vi "visadenemesi_max30100.vi"() -> ()   [LabVIEW 2017]
uses:
  <vilib>/Instr/_visa.llb/VISA Configure Serial Port (Instr).vi
panel:
  in  "stop":bool
  out "Numeric":dbl
  out "Thermometer":dbl(slide) scale=0.0..100.0
  in  "VISA resource name":refnum<visa-resource-name>
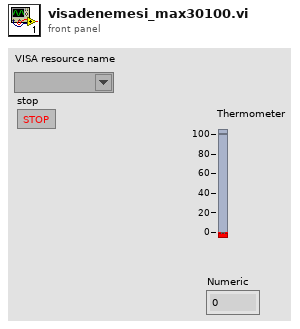
[diagram p1: front panel]
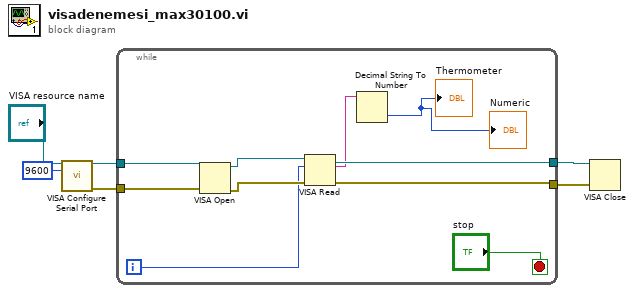
[diagram p0: block diagram]
diagram:
  n1 = call-poly "VISA Configure Serial Port"("VISA resource name"="VISA resource name", "baud rate (9600)"=u32 9600) -> ("VISA resource name out"=w2:refnum<visa-resource-name>, "error out"=w5:errorcluster)  [unwired: 12 in]
  n2 = while {
    tunnel: w5 -> [w16]
    tunnel: [w14] -> w4
    tunnel: [w13] -> w3
    tunnel: w2 -> [w11]
    i -> [w9]
    stop <- "stop" stop-if-true
    n3 = VISA Open(error in (no error)=w16, VISA resource name=w11) -> (VISA resource name=w12:refnum<visa-resource-name>, error out=w15:errorcluster)  [unwired: 3 in]
    n4 = VISA Read(VISA resource name=w12, byte count=w9, error in (no error)=w15) -> (VISA resource name out=w13:refnum<visa-resource-name>, read buffer=w10:string, error out=w14:errorcluster)  [unwired: 1 out]
    n5 = Decimal String To Number(string=w10) -> (number=→"Thermometer" →"Numeric":i32)  [unwired: 2 in, 1 out]
  }
  n6 = VISA Close(VISA resource name=w3, error in (no error)=w4) -> ()  [unwired: 1 out]
